vi "EPEC_Process.vi"(8 "error in":errorcluster, 11 "PublicMessage":refnum<user-event>) -> (0 "error out":errorcluster)   [LabVIEW 2014]
doc: "This is EventStateMachine.\nThis is a part of EPEC framework.\n\nUse private event to communicate with only this module.\nUse public event to communicate to all and receive from all module.\n\nIf you need to communicate with specific ESM only share event external or by FGV."
panel:
  in  "stop":bool
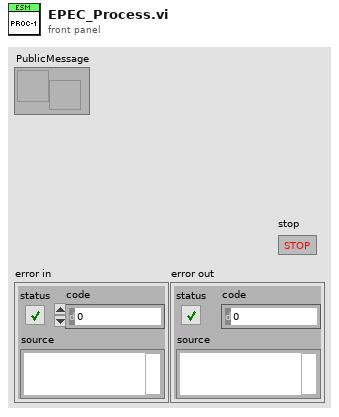
[diagram p1: front panel]
types:
  T1 = cluster{"PublicMessage":refnum<user-event>, "PrivateMessage":refnum<user-event>}
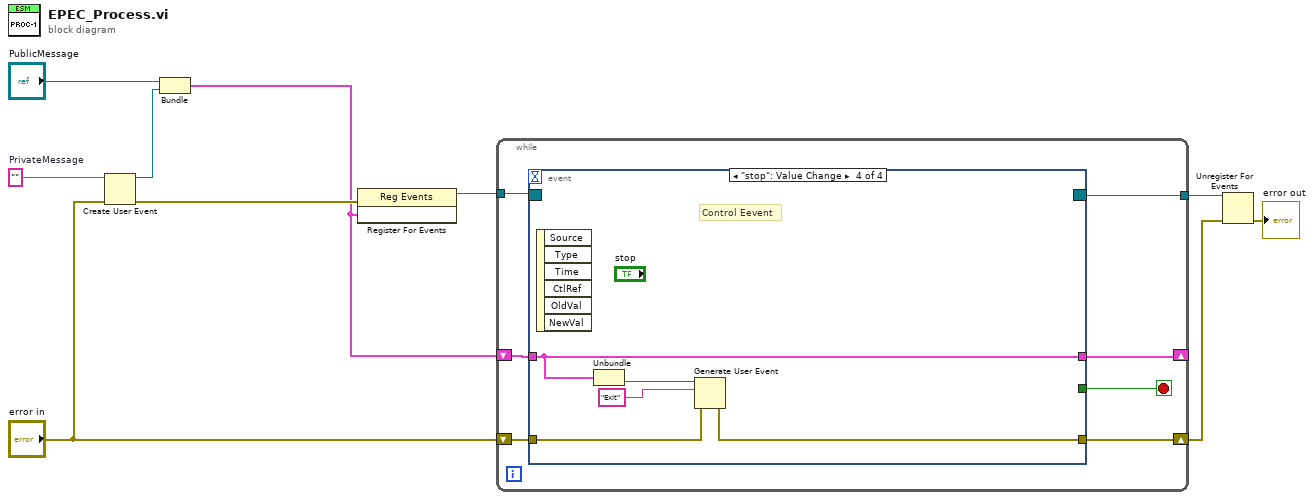
[diagram p0: block diagram]
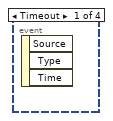
[diagram p2: hidden frame]
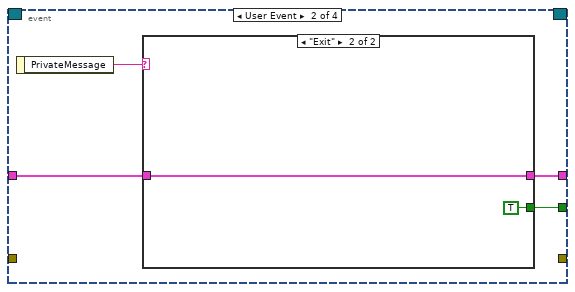
[diagram p3: hidden frame]
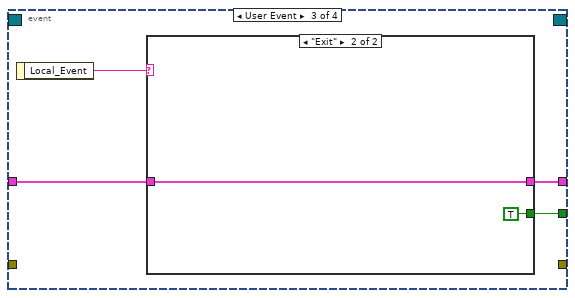
[diagram p5: hidden frame]
diagram:
  w8 = ""  # PrivateMessage
  n1 = Create User Event(user event datatype=w8, error in="error in") -> (user event=w5:refnum<user-event>, error out=w9:errorcluster)
  n2 = Bundle("PublicMessage"="PublicMessage", "PrivateMessage"=w5) -> (w7:T1)  [unwired: 1 in]
  n3 = register-events(error in=w9, w7) -> (reference out=w10:refnum<event-registration>)  [unwired: 1 in, 1 out]
  n4 = while {
    tunnel: w10 -> [w17]
    shift-right: [w15] -> _
    shift-left: w7 -> [w16]
    shift-right: [w12] -> w3
    shift-left: "error in" -> [w13]
    tunnel: [w11] -> w4
    stop <- w14 stop-if-true
    n5 = event shown="[3] \"stop\": Value Change" {
      selector: w17 -> [_ _ _ _]
      dyn-events: [_ _ _ _] -> w11
      timeout: _ -> [_ _ _ _]
      tunnel: w16 -> [_ w19 w26 w34]
      tunnel: [_ w18 w25 w34] -> w15
      tunnel: [_ w21 w28 _] -> w14
      tunnel: w13 -> [_ _ _ w33]
      tunnel: [_ _ _ w32] -> w12
      event Timeout {
        n6 = event-data() -> ()  [unwired: 1 in, 3 out]
      }
      event User Event {
        n7 = event-data() -> ("PrivateMessage"=w20:string)  [unwired: 1 in]
        n8 = case shown="\"Exit\"" w20 {
          tunnel: [_ TRUE] -> w21
          tunnel: w19 -> [w22 w23]
          tunnel: [w22 w23] -> w18
          frame "False", Default {
          }
          frame "Exit" {
          }
        }
      }
      event User Event {
        n9 = event-data() -> ("Local_Event"=w27:string)  [unwired: 1 in]
        n10 = case shown="\"Exit\"" w27 {
          tunnel: [_ TRUE] -> w28
          tunnel: w26 -> [w29 w30]
          tunnel: [w29 w30] -> w25
          frame "False", Default {
          }
          frame "Exit" {
          }
        }
      }
      event "stop": Value Change {
        # "Control Eevent"
        n11 = event-data() -> ()  [unwired: 1 in, 6 out]
        n12 = Unbundle(w34) -> ("PrivateMessage"=w35:refnum<user-event>)  [unwired: 1 out]
        n13 = Generate User Event(user event=w35, event data cluster="Exit", error in=w33) -> (error out=w32:errorcluster)  [unwired: 1 in, 1 out]
      }
    }
  }
  n14 = Unregister For Events(event registration refnum=w4, error in=w3) -> (error out=→"error out":errorcluster)
